vi "Fit Description.vi"(8 "error in (no error)":errorcluster, 9 "Word Wrap Bound":u32=482, 10 "Description":string, 11 "Project Information":string="More Information") -> (0 "error out":errorcluster, 1 "Description out":string, 2 "End of Desc Character":i32, 3 "Tail Pos":u32)   [LabVIEW 2021]
panel:
  in  "Local Temp Var":string
  in  "Line number":u8=2
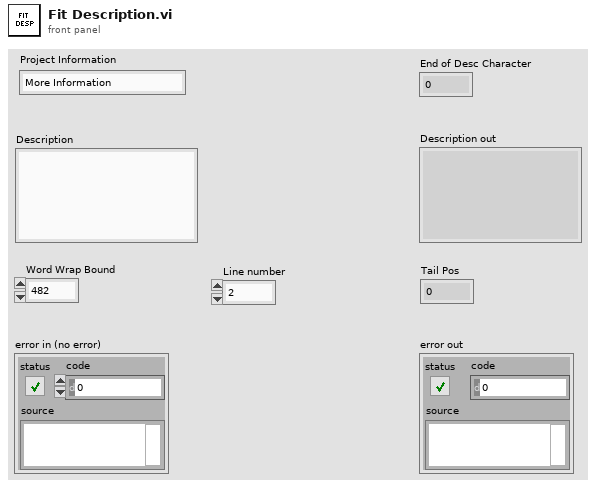
[diagram p1: front panel]
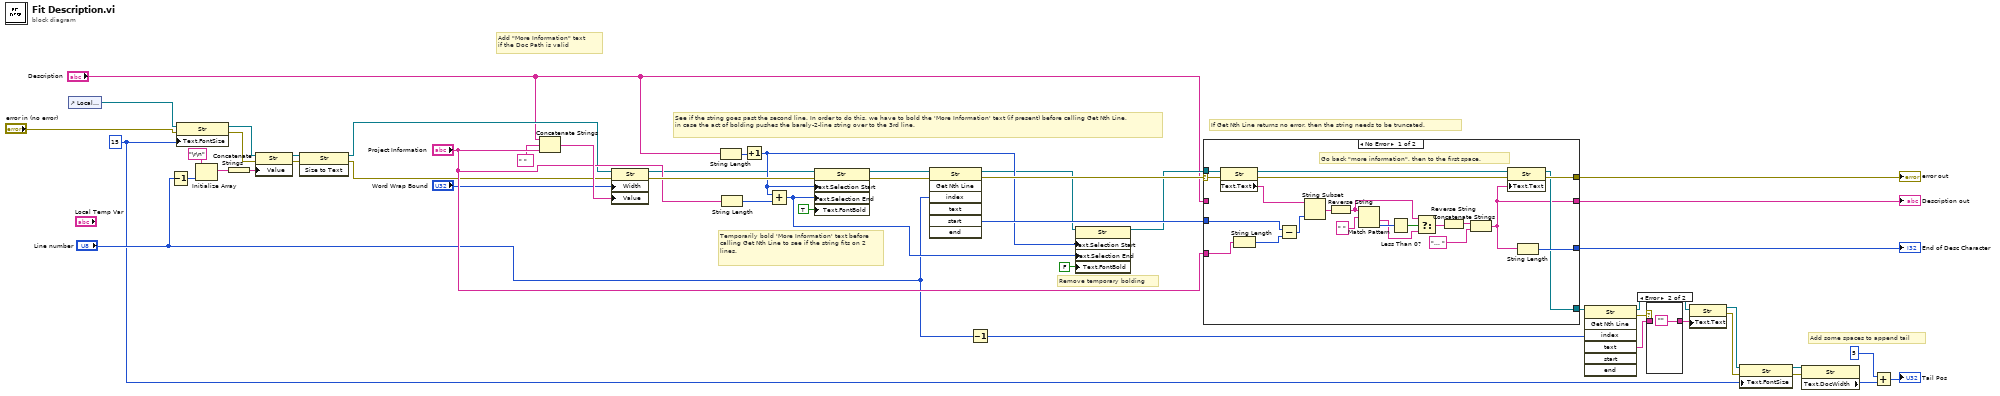
[diagram p0: block diagram]
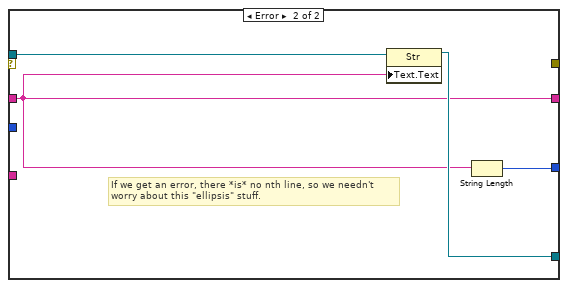
[diagram p3: hidden frame]
diagram:
  w8 = u32 15 ("Text.Font:Size")
  # "Add some spaces to append tail"
  # "Remove temporary bolding"
  # "Temporarily bold 'More Information' text before calling Get Nth Line to see if the string fits on 2 lines."
  # "If Get Nth Line returns no error, then the string needs to be truncated."
  # "See if the string goes past the second line. In order to do this, we have to bold the 'More Information' text (if present) before calling Get Nth Line, in case the act of bolding pushes the barely-2-line string over to the 3rd line."
  # "Add \"More Information\" text\nif the Doc Path is valid"
  n1 = control-ref of="Local Temp Var"() -> (w18:refnum<vi>)
  n2 = Decrement(x="Line number") -> (x-1=w43:u8)
  n3 = property on="Property Node" class="Str"(reference=w18, error in="error in (no error)", "Text.FontSize"=w8) -> (reference out=w34:refnum<vi>, error out=w42:errorcluster)
  n4 = Initialize Array("\r\n", w43) -> (w46:string[])
  n5 = Concatenate Strings(w46) -> (w45:string)
  n6 = property on="Property Node" class="Str"(reference=w34, error in=w42, "Value"=w45) -> (reference out=w35:refnum<vi>, error out=w44:errorcluster)
  n7 = invoke on="Invoke Node" class="Str" method="Size to Text"(reference=w35, error in=w44) -> (reference out=w29:refnum<vi>, error out=w22:errorcluster)  [unwired: 1 in, 1 out]
  n8 = Concatenate Strings("Description", " ", "Project Information") -> (w48:string)
  n9 = property on="Property Node" class="Str"(reference=w29, error in=w22, "Width"="Word Wrap Bound", "Value"=w48) -> (reference out=w33:refnum<vi>, error out=w41:errorcluster)
  n10 = String Length(string="Description") -> (length=w27:i32)
  n11 = String Length(string="Project Information") -> (length=w26:i32)
  n12 = Increment(x=w27) -> (x+1=w37:i32)
  n13 = Add(x=w37, y=w26) -> (x+y=w36:i32)
  n14 = property on="Property Node" class="Str"(reference=w33, error in=w41, "Text.Selection Start"=w37, "Text.Selection End"=w36, "Text.FontBold"=TRUE ("Text.Font:Bold")) -> (reference out=w32:refnum<vi>, error out=w40:errorcluster)
  n15 = invoke on="Invoke Node" class="Str" method="Get Nth Line"(reference=w32, error in=w40, "index"="Line number") -> (reference out=w31:refnum<vi>, error out=w49:errorcluster, "start"=w38:u32)  [unwired: 4 in, 4 out]
  n16 = Decrement(x="Line number") -> (x-1=w16:u8)
  n17 = property on="Property Node" class="Str"(reference=w31, "Text.Selection Start"=w37, "Text.Selection End"=w36, "Text.FontBold"=FALSE ("Text.Font:Bold")) -> (reference out=w30:refnum<vi>)  [unwired: 1 in, 1 out]
  n18 = case shown="No Error" w49 {
    selector: w49 -> [w70 _]
    tunnel: w38 -> [w71 _]
    tunnel: [w66 _] -> w19
    tunnel: "Project Information" -> [w67 _]
    tunnel: [w51 w72] -> w20
    tunnel: [w65 w75] -> w21
    tunnel: "Description" -> [_ w72]
    tunnel: w30 -> [w64 w73]
    tunnel: [w54 w74] -> w15
    frame No Error {
      # "Go back \"more information\", then to the first space."
      n19 = property on="Property Node" class="Str"(reference=w64, error in=w70) -> (reference out=w63:refnum<vi>, error out=w68:errorcluster, "Text.Text"=w69:string)
      n20 = String Length(string=w67) -> (length=w50:i32)
      n21 = Subtract(x=w71, y=w50) -> (x-y=w62:u32)
      n22 = String Subset(string=w69, length (rest)=w62) -> (substring=w60:string)  [unwired: 1 in]
      n23 = Reverse String(1:w60) -> (0:w57:string)
      n24 = Match Pattern(string=w57, regular expression=" ") -> (after substring=w55:string, offset past match=w59:i32)  [unwired: 1 in, 2 out]
      n25 = Less Than 0?(x=w59) -> (x < 0?=w58:bool)
      n26 = Select(t=w57, s=w58, f=w55) -> (s? t:f=w56:string)
      n27 = Reverse String(1:w56) -> (0:w53:string)
      n28 = Concatenate Strings(w53, "... ") -> (w51:string)
      n29 = property on="Property Node" class="Str"(reference=w63, error in=w68, "Text.Text"=w51) -> (reference out=w54:refnum<vi>, error out=w66:errorcluster)
      n30 = String Length(string=w51) -> (length=w65:i32)
    }
    frame Error {
      # "If we get an error, there *is* no nth line, so we needn't worry about this \"ellipsis\" stuff."
      n31 = property on="Property Node" class="Str"(reference=w73, "Text.Text"=w72) -> (reference out=w74:refnum<vi>)  [unwired: 1 in, 1 out]
      n32 = String Length(string=w72) -> (length=w75:i32)
    }
  }
  "End of Desc Character" <- w21
  "Description out" <- w20
  "error out" <- w19
  n33 = invoke on="Invoke Node" class="Str" method="Get Nth Line"(reference=w15, "index"=w16) -> (reference out=w3:refnum<vi>, error out=w11:errorcluster, "text"=w10:string)  [unwired: 5 in, 4 out]
  n34 = case shown="Error" w11 {
    tunnel: w10 -> [w76 _]
    tunnel: [w76 ""] -> w7
    frame No Error {
    }
    frame Error {
    }
  }
  n35 = property on="Property Node" class="Str"(reference=w3, "Text.Text"=w7) -> (reference out=w2:refnum<vi>, error out=w12:errorcluster)  [unwired: 1 in]
  n36 = property on="Property Node" class="Str"(reference=w2, error in=w12, "Text.FontSize"=w8) -> (reference out=w1:refnum<vi>, error out=w13:errorcluster)
  n37 = property on="Property Node" class="Str"(reference=w1, error in=w13) -> ("Text.DocWidth"=w5:u32)  [unwired: 2 out]
  n38 = Add(x=u32 5, y=w5) -> (x+y=→"Tail Pos":u32)
